vi "temp.vi"() -> ()   [LabVIEW 2017]
uses:
  Error Handler/Controls/Error Data.ctl
  Error Handler/Controls/Error Level.ctl
  Configuration/Controls/Config Record.ctl
  Configuration/Controls/Config Data.ctl
  Configuration/Controls/Config Command.ctl
  Views/Vehicle Position View/Controls/Vehicle - Station Slider.ctl
  Controller/Controls/Controller - Wash Step.ctl
  Views/Entry Console View/Controls/Entry Console - Wash Steps.ctl
panel:
  in  "Wash Step Start":refnum<user-event>
  in  "Vehicle Out of Position":refnum<user-event>
  in  "Wash Cycle Start":refnum<user-event>
  in  "Wash Cycle Complete":refnum<user-event>
  in  "Wash Step Complete":refnum<user-event>
  in  "Wash Step Start":refnum<user-event>
  in  "Wash Step Exec":refnum<user-event>
  in  "Wash Sequence":refnum<data-value>
  in  "Station":refnum<user-event>
  in  "Config Lock DVR":refnum<data-value>
  in  "Config Lock":refnum<user-event>
  in  "Config Data":refnum<user-event>
  in  "Config Records DVR":refnum<data-value>
  in  "Error":refnum<user-event>
  in  "Stop DVR":refnum<data-value>
  in  "Stop":refnum<user-event>
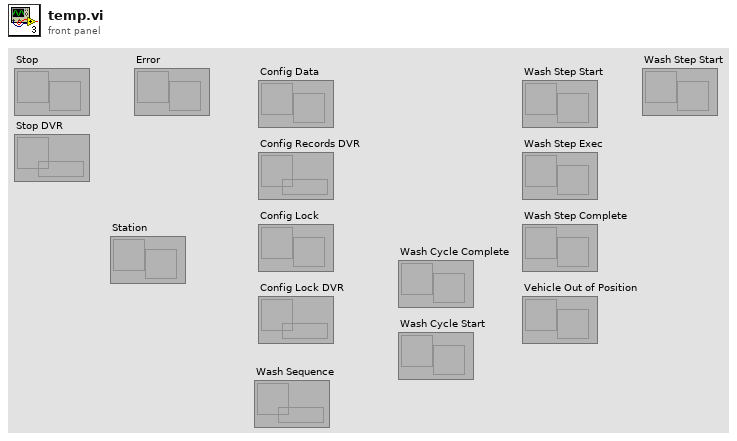
[diagram p1: front panel]
types:
  T1 = typedef "Entry Console - Wash Steps.ctl" = cluster{"Under Body Wash":bool, "Bug Remover":bool, "Pre-Soak":bool, "High Pressure Wash":bool, "Low Pressure Wax":bool, "Spot Free Rinse":bool, "Tire Shine Foam":bool, "Air Dry":bool}
  T2 = typedef "Controller - Wash Step.ctl" = enum16{"Under Body Wash", "Bug Remover", "Pre-Soak", "High Pressure Wash", "Low Pressure Wax", "Spot Free Rinse", "Tire Shine Foam", "Air Dry"}
  T3 = typedef "Vehicle - Station Slider.ctl" = u8
  T4 = typedef "Config Data.ctl" = cluster{"Config Command":T5, "Data":variant}
  T5 = typedef "Config Command.ctl" = enum16{"Read", "Query", "Insert", "Update"}
  T6 = typedef "Config Record.ctl" = cluster{"Wash Step":string, "Station":string, "Step Duration":u32}
  T7 = typedef "Error Data.ctl" = cluster{"Error Level":T8, "Data":variant}
  T8 = typedef "Error Level.ctl" = enum16{"Minor Error", "Wash Cycle Error", "System Error"}
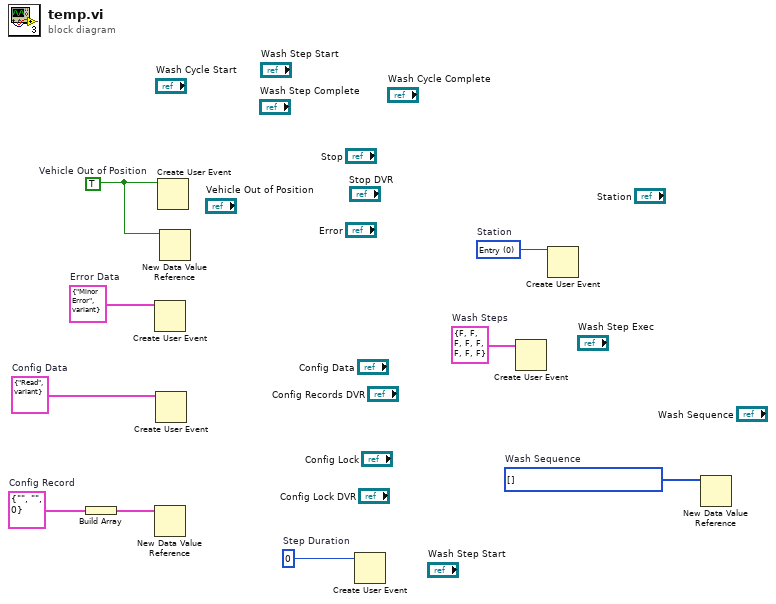
[diagram p0: block diagram]
diagram:
  w1 = u32 0  # Step Duration
  w2 = T1 {"Under Body Wash"=FALSE, "Bug Remover"=FALSE, "Pre-Soak"=FALSE, "High Pressure Wash"=FALSE, "Low Pressure Wax"=FALSE, "Spot Free Rinse"=FALSE, "Tire Shine Foam"=FALSE, "Air Dry"=FALSE}  # Wash Steps
  w3 = T2[] [] items=["Under Body Wash", "Bug Remover", "Pre-Soak", "High Pressure Wash", "Low Pressure Wax", "Spot Free Rinse", "Tire Shine Foam", "Air Dry"]  # Wash Sequence
  w4 = T3 0 items=["Entry", "Station1", "Station2", "Station3", "Exit"]  # Station
  w5 = T4 {"Config Command"=enum."Read", "Data"=variant}  # Config Data
  w7 = T6 {"Wash Step"="", "Station"="", "Step Duration"=0}  # Config Record
  w8 = T7 {"Error Level"=enum."Minor Error", "Data"=variant}  # Error Data
  w9 = TRUE  # Vehicle Out of Position
  n1 = Build Array(w7) -> (w6:T6[])
  n2 = Create User Event(user event datatype=w8) -> ()  [unwired: 1 in, 2 out]
  n3 = New Data Value Reference(data value=w6) -> ()  [unwired: 1 in, 2 out]
  n4 = Create User Event(user event datatype=w5) -> ()  [unwired: 1 in, 2 out]
  n5 = Create User Event(user event datatype=w9) -> ()  [unwired: 1 in, 2 out]
  n6 = New Data Value Reference(data value=w9) -> ()  [unwired: 1 in, 2 out]
  n7 = Create User Event(user event datatype=w1) -> ()  [unwired: 1 in, 2 out]
  n8 = Create User Event(user event datatype=w2) -> ()  [unwired: 1 in, 2 out]
  n9 = Create User Event(user event datatype=w4) -> ()  [unwired: 1 in, 2 out]
  n10 = New Data Value Reference(data value=w3) -> ()  [unwired: 1 in, 2 out]
